vi "Fixed Valve Control.vi"(7 "Fixed  Valve Control":T1, 8 "Error In":errorcluster, 9 "GEA Inputs":T2 {"Destination" format="%.0x"; "Source" format="%.0x"}, 10 "Standalone?":bool, 11 "GEA2 Reference In":refnum<k24>) -> (0 "Error Out":errorcluster, 3 "GEA2 Reference Out":refnum<k24>)   [LabVIEW 2016, in "TL27.lvlib"]
uses:
  Projects/TL27.lvlib
  C:/Automation/DLLs/PC Dot Net/GeaCommunication.dll
  Common/LabVIEW GEA2 Toolkit/LabVIEW_GEA2_Toolkit.lvlibp/type defs/Source_Destination.ctl
  type defs/Fixed Valve Control.ctl
  Common/LabVIEW GEA2 Toolkit/LabVIEW_GEA2_Toolkit.lvlibp/type defs/ERD Write Data In.ctl
  Common/LabVIEW GEA2 Toolkit/LabVIEW_GEA2_Toolkit.lvlibp/type defs/Data Type.ctl
  Common/LabVIEW GEA2 Toolkit/LabVIEW_GEA2_Toolkit.lvlibp
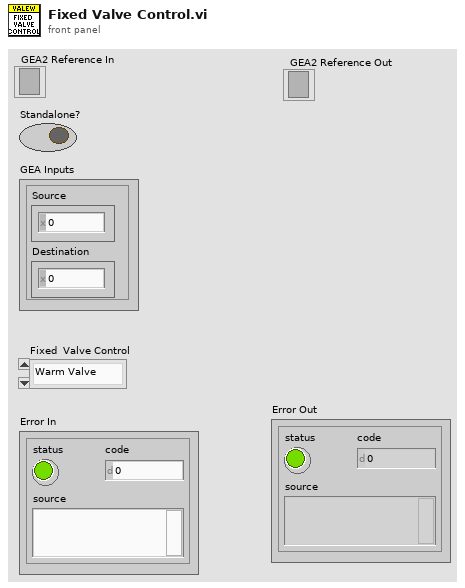
[diagram p1: front panel]
types:
  T1 = typedef "TL27.lvlib/Fixed Valve Control.ctl" = enum16{"Warm Valve", "Hot Valve", "Cold Valve"}
  T2 = typedef "LabVIEW_GEA2_Toolkit.lvlibp/Source_Destination.ctl" = cluster{"Source":u8, "Destination":u8}
  T3 = typedef "LabVIEW_GEA2_Toolkit.lvlibp/ERD Write Data In.ctl" = cluster{"ERD Number":u16, "Data Type":T4, "Data":string}
  T4 = typedef "LabVIEW_GEA2_Toolkit.lvlibp/Data Type.ctl" = enum16{"string", "boolean", "uint8_t", "uint16_t", "uint32_t", "uint64_t", "int8_t", "int16_t", "int32_t", "int64_t"}
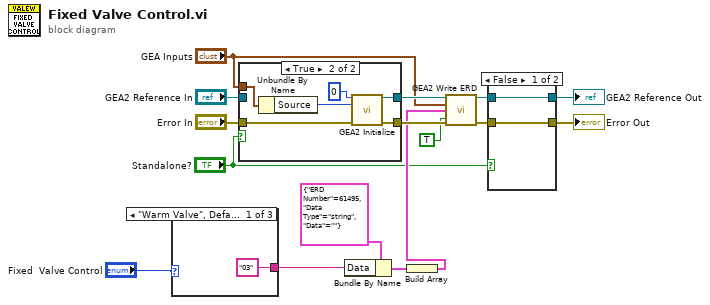
[diagram p0: block diagram]
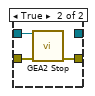
[diagram p2: hidden frame]
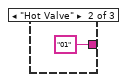
[diagram p4: hidden frame]
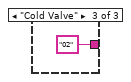
[diagram p5: hidden frame]
diagram:
  n1 = case shown="\"Warm Valve\", Default" "Fixed  Valve Control" {
    tunnel: ["03" "01" "02"] -> w7
    frame "Warm Valve", Default {
    }
    frame "Hot Valve" {
    }
    frame "Cold Valve" {
    }
  }
  n2 = case shown="True" "Standalone?" {
    tunnel: "Error In" -> [w20 w27]
    tunnel: [w20 w26] -> w16
    tunnel: "GEA2 Reference In" -> [w21 _]
    tunnel: [w21 w25] -> w11
    tunnel: "GEA Inputs" -> [_ w23]
    frame False {
    }
    frame True {
      n3 = Unbundle By Name(w23) -> ("Source"=w24:u8)
      n4 = call "GEA2 Initialize.vi"("Board Index"=0, "Source Address"=w24, "error in"=w27) -> ("GEA2 Reference Out"=w25:refnum<k24>, "error out"=w26:errorcluster)  [unwired: 10 in, 1 out]
    }
  }
  n5 = Bundle By Name(cluster=T3 {"ERD Number"=61495, "Data Type"=enum."string", "Data"=""} ("ERD Write Data In"), "Data"=w7) -> (w9:T3)
  n6 = Build Array(w9) -> (w8:T3[])
  n7 = call "GEA2 Write ERD.vi"("GEA2 Reference In"=w11, "GEA Inputs"="GEA Inputs", "Write ERD List"=w8, "Error In"=w16, "Verify ERD Response?"=TRUE) -> ("GEA2 Reference Out"=w3:refnum<k24>, "Error Out"=w2:errorcluster)  [unwired: 8 in, 1 out]
  n8 = case shown="False" "Standalone?" {
    tunnel: w2 -> [w28 w32]
    tunnel: [w28 w31] -> w14
    tunnel: w3 -> [w29 w30]
    tunnel: [w29 _] -> w12
    frame False {
    }
    frame True {
      n9 = call "GEA2 Stop.vi"("GEA2 Reference In"=w30, "Error In"=w32) -> ("Error Out"=w31:errorcluster)  [unwired: 13 in]
    }
  }
  "Error Out" <- w14
  "GEA2 Reference Out" <- w12
